vi "m1m3_acceptCommand_ProgramILC.vi"(8 "error in (no error)":errorcluster, 11 "command_ProgramILC_Ctl":T1={"ActuatorId"=0, "FilePath"="                                                                                                                                                                                                                                                                "}) -> (0 "error out":errorcluster, 2 "function return":i32, 3 "command_ProgramILC_Ctl out":T1={"ActuatorId"=0, "FilePath"="                                                                                                                                                                                                                                                                "})   [LabVIEW 2016, in "SALLV_m1m3.lvlib"]
doc: "int m1m3_shm_acceptCommand_ProgramILCLV(m1m3_command_ProgramILCLV *command_ProgramILC_Ctl );"
uses:
  SALLV_m1m3.lvlib
  DataTypes/command_ProgramILC.ctl
  SALLV_m1m3.so
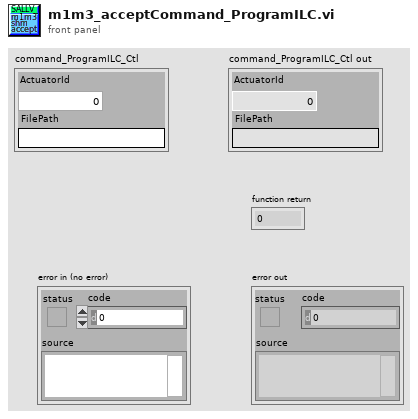
[diagram p1: front panel]
types:
  T1 = typedef "SALLV_m1m3.lvlib/command_ProgramILC.ctl" = cluster{"ActuatorId":i32, "FilePath":string}
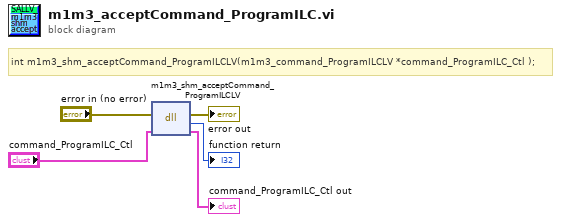
[diagram p0: block diagram]
diagram:
  # "int m1m3_shm_acceptCommand_ProgramILCLV(m1m3_command_ProgramILCLV *command_ProgramILC_Ctl );"
  n1 = dll-call lib="opt/CODE/SALLV_m1m3/SALLV_m1m3.*" fn="m1m3_shm_acceptCommand_ProgramILCLV"(error in="error in (no error)", "command_ProgramILC_Ctl"="command_ProgramILC_Ctl") -> (error out=→"error out":errorcluster, →"function return":i32, "command_ProgramILC_Ctl"=→"command_ProgramILC_Ctl out":T1)  [unwired: 2 in, 1 out]
